vi "AlignControlSelection.vi"(6 "Error terminals":T1, 8 "error in (no error)":errorcluster, 9 "Item to enclose in case structure":refnum<vi>[](array[refnum]), 10 "Control terminals on top-level":refnum<vi>[](array[refnum]), 11 "VI in":refnum<vi>) -> (0 "error out":errorcluster, 1 "Item to enclose in case structure (dup)":refnum<vi>[](array[refnum]), 3 "VI out (dup)":refnum<vi>)   [LabVIEW 2017, in "ErrorStructureDrawer.lvlib"]
doc: "Seperates a list of controls into controls and indicators, and then aligns and moves each of those two groups seperately. They are moved in order to make space for the new case structure."
uses:
  ErrorStructureDrawer.lvlib
  Controls/ErrorTerminals.ctl
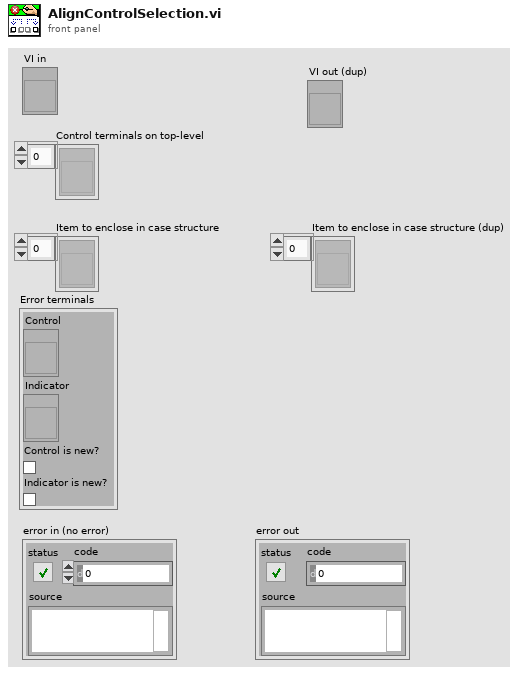
[diagram p1: front panel]
types:
  T1 = typedef "ErrorStructureDrawer.lvlib/ErrorTerminals.ctl" = cluster{"Control":refnum<vi>, "Indicator":refnum<vi>, "Control is new?":bool, "Indicator is new?":bool}
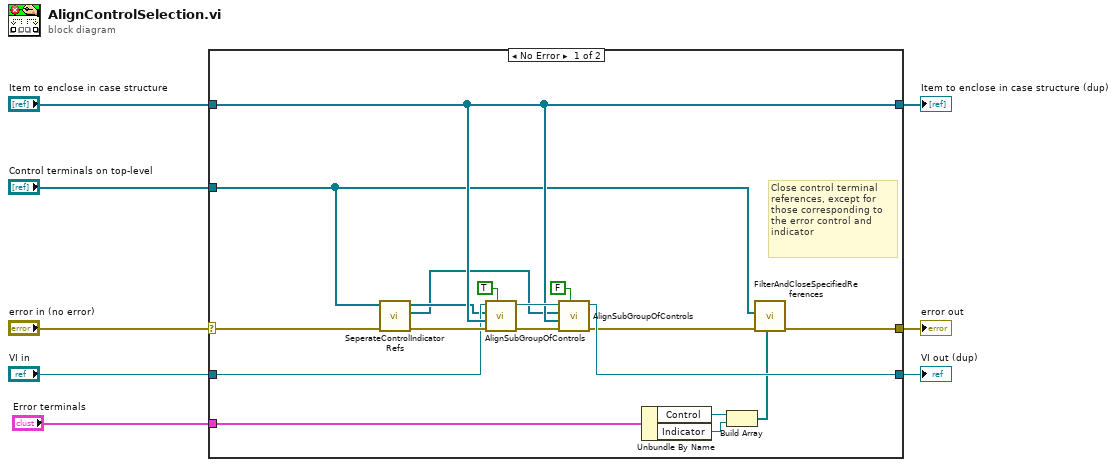
[diagram p0: block diagram]
diagram:
  n1 = case shown="No Error" "error in (no error)" {
    selector: "error in (no error)" -> [w21 w28]
    tunnel: "VI in" -> [w19 w27]
    tunnel: "Item to enclose in case structure" -> [w22 w29]
    tunnel: "Control terminals on top-level" -> [w10 _]
    tunnel: [w11 w28] -> w5
    tunnel: [w22 w29] -> w4
    tunnel: [w18 w27] -> w2
    tunnel: "Error terminals" -> [w9 _]
    frame No Error {
      # "Close control terminal references, except for those corresponding to the error control and indicator"
      n2 = call "SeperateControlIndicatorRefs.vi"("error in (no error)"=w21, "Terminal references"=w10) -> ("error out"=w20:errorcluster, "Indicator references"=w16:refnum<vi>[], "Control references"=w17:refnum<vi>[])  [unwired: 7 in]
      n3 = call "AlignSubGroupOfControls.vi"("Controls [t] / indicators [f]"=TRUE, "error in (no error)"=w20, "Case structure contents to move away from"=w22, "Controls to align and move"=w17, "VI in"=w19) -> ("error out"=w26:errorcluster, "VI ref (dup)"=w23:refnum<vi>)  [unwired: 5 in]
      n4 = call "AlignSubGroupOfControls.vi"("Controls [t] / indicators [f]"=FALSE, "error in (no error)"=w26, "Case structure contents to move away from"=w22, "Controls to align and move"=w16, "VI in"=w23) -> ("error out"=w12:errorcluster, "VI ref (dup)"=w18:refnum<vi>)  [unwired: 5 in]
      n5 = Unbundle By Name(w9) -> ("Control"=w15:refnum<vi>, "Indicator"=w13:refnum<vi>)
      n6 = Build Array(w15, w13) -> (w14:refnum<vi>[])
      n7 = call "FilterAndCloseSpecifiedReferences.vi"("Control references to filter"=w14, "error in (no error)"=w12, "Control references to close"=w10) -> ("error out"=w11:errorcluster)  [unwired: 8 in]
    }
    frame Error {
    }
  }
  "error out" <- w5
  "VI out (dup)" <- w2
  "Item to enclose in case structure (dup)" <- w4
